vi "LinearFilter_Factorial.vi"(11 "N":i32) -> (3 "Factorial":dbl)   [LabVIEW 2019, in "Trajectory_Library.lvlib"]
doc: "Computes the factorial of \"n\". This is an internal function.\n\n\nInputs: \n - n - Integer value >= 1.\n\nOutputs:\n - factorial - The calculated factorial value, as an integer."
uses:
  Trajectory_Library.lvlib
  <vilib>/gmath/NI_Gmath.lvlib
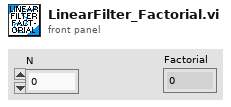
[diagram p1: front panel]
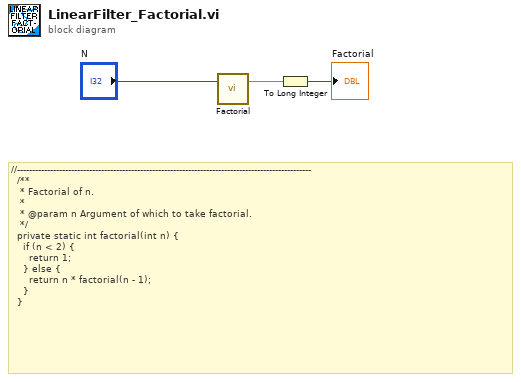
[diagram p0: block diagram]
diagram:
  # "//--------------------------------------------------------------------------------------------------\n  /**\n   * Factorial of n.\n   *\n   * @param n Argument of which to take factorial.\n   */\n  private static int factorial(int n) {\n    if (n < 2) {\n      return 1;\n    } else {\n      return n * factorial(n - 1);\n    }\n  }"
  n1 = call <vilib>:"Factorial.vi"("n"="N") -> ("n!"=w2:dbl)  [unwired: 2 in]
  n2 = To Long Integer(number=w2) -> (32bit integer=→"Factorial":i32)
